vi "deleteme2.vi"(8 "error in (no error)":errorcluster, 11 "WaveformProcessor in":refnum<class "WaveformProcessor.lvclass">) -> (0 "error out":errorcluster, 3 "WaveformProcessor out":refnum<class "WaveformProcessor.lvclass">)   [LabVIEW 2019, in "Variant Parser.lvlib" / "WaveformProcessor.lvclass"]
uses:
  Library/WaveformProcessor.lvclass
  Custom Controls/Pulse Analysis.ctl
  Library/WaveformProcessor.lvclass/WaveformProcessor.ctl
panel:
  out "MissingChannel":bool
  out "MissingPulse":bool
  out "PulseAnalysis":T1[](array[typedef])
  in  "Target Channel":string
  in  "Pulse Count (1)":i32=1
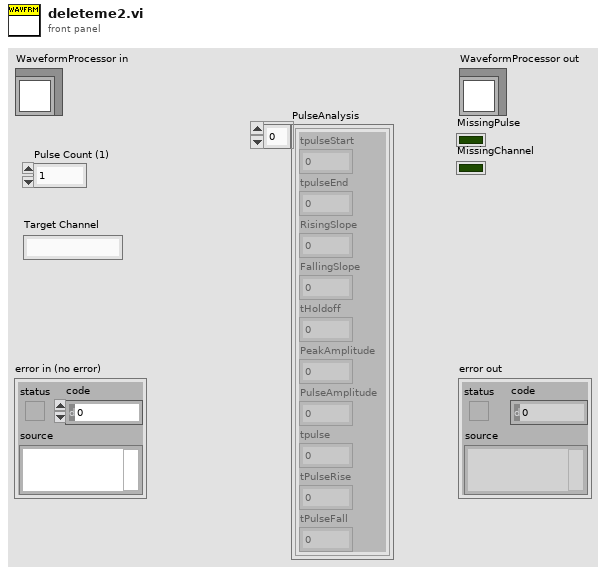
[diagram p1: front panel]
types:
  T1 = typedef "Variant Parser.lvlib/WaveformProcessor.lvclass/Pulse Analysis.ctl" = cluster{"tpulseStart":dbl, "tpulseEnd":dbl, "RisingSlope":dbl, "FallingSlope":dbl, "tHoldoff":dbl, "PeakAmplitude":dbl, "PulseAmplitude":dbl, "tpulse":dbl, "tPulseRise":dbl, "tPulseFall":dbl}
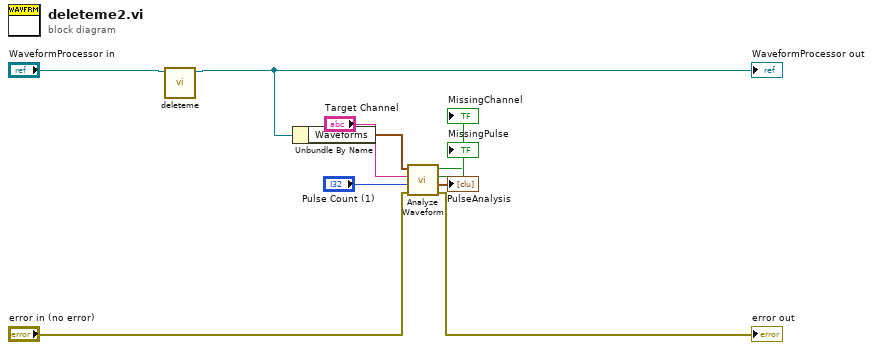
[diagram p0: block diagram]
diagram:
  n1 = call "deleteme.vi"("WaveformProcessor in"="WaveformProcessor in") -> ("WaveformProcessor out"=w9:refnum<class "WaveformProcessor.lvclass">)  [unwired: 9 in, 1 out]
  "WaveformProcessor out" <- w9
  n2 = Unbundle By Name(w9) -> ("Waveforms"=w8:waveform(dbl)[])
  n3 = call "Analyze Waveform.vi"("error in (no error)"="error in (no error)", "Pulse Count (1)"="Pulse Count (1)", "Target Channel"="Target Channel", "CapturedData"=w8) -> ("error out"=→"error out":errorcluster, "PulseAnalysis"=→"PulseAnalysis":T1[], "MissingPulse"=→"MissingPulse":bool, "MissingChannel"=→"MissingChannel":bool)  [unwired: 4 in]
